vi "Create Image Name.vi"(8 "error in (no error)":errorcluster, 11 "Save Image in":refnum<class "Save Image.lvclass">) -> (0 "error out":errorcluster, 3 "Save Image out":refnum<class "Save Image.lvclass">)   [LabVIEW 2018, in "Save Image.lvclass"]
uses:
  Save Image.lvclass
  Save Image.lvclass/Save Image.ctl
  Simulated_Header/Simulated_Header.lvclass
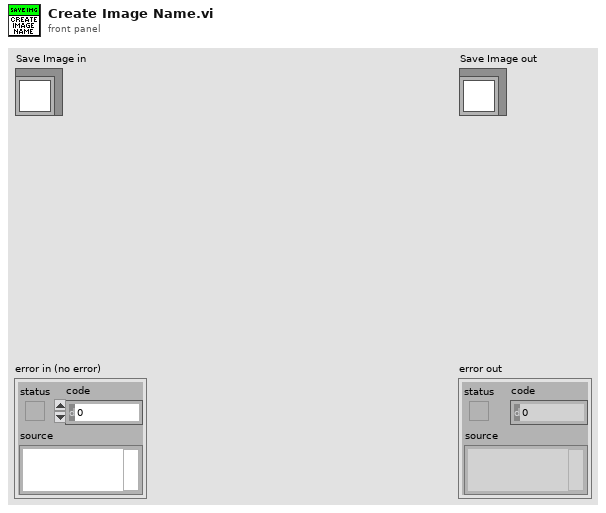
[diagram p1: front panel]
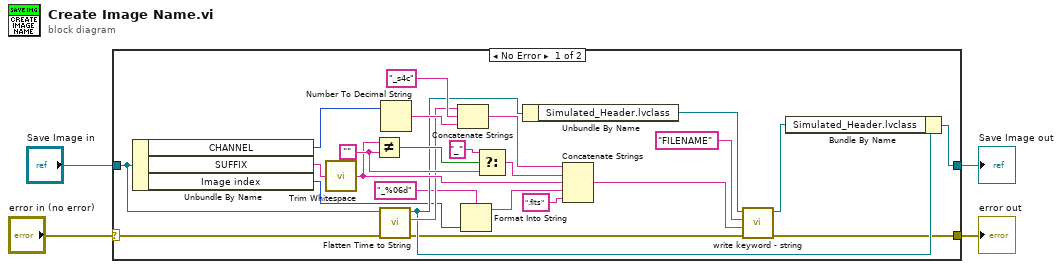
[diagram p0: block diagram]
diagram:
  n1 = case shown="No Error" "error in (no error)" {
    selector: "error in (no error)" -> [w18 w31]
    tunnel: [w9 w31] -> w3
    tunnel: [w15 w30] -> w1
    tunnel: "Save Image in" -> [w17 w30]
    frame No Error {
      w23 = ""
      n2 = Unbundle By Name(w17) -> ("CHANNEL"=w20:u16, "SUFFIX"=w22:string, "Image index"=w13:u32)
      n3 = call <vilib>:"Trim Whitespace.vi"("string"=w22) -> ("trimmed string"=w21:string)  [unwired: 1 in]
      n4 = Not Equal?(x=w21, y=w23) -> (x != y?=w26:bool)
      n5 = call "Flatten Time to String.vi"("error in (no error)"=w18, "Save Image in"=w17) -> ("error out"=w8:errorcluster, "flattened string"=w19:string, "Save Image out"=w16:refnum<class "Save Image.lvclass">)  [unwired: 7 in]
      n6 = Number To Decimal String(number=w20) -> (decimal integer string=w28:string)  [unwired: 1 in]
      n7 = Concatenate Strings(w19, "_s4c" ("string"), w28) -> (w27:string)
      n8 = Format Into String(format string="_%06d", w13) -> (resulting string=w12:string)  [unwired: 2 in, 1 out]
      n9 = Select(t="_" ("string"), s=w26, f=w23) -> (s? t:f=w24:string)
      n10 = Unbundle By Name(w16) -> ("Simulated_Header.lvclass"=w7:refnum<class "Simulated_Header.lvclass">)
      n11 = Concatenate Strings(w27, w24, w21, w12, ".fits" ("string")) -> (w6:string)
      n12 = call "write keyword - string.vi"("error in (no error)"=w8, "value"=w6, "keyword"="FILENAME", "Simulated_Header in"=w7) -> ("error out"=w9:errorcluster, "Simulated_Header out"=w10:refnum<class "Simulated_Header.lvclass">)  [unwired: 6 in]
      n13 = Bundle By Name(cluster=w16, "Simulated_Header.lvclass"=w10) -> (w15:refnum<class "Save Image.lvclass">)
    }
    frame Error {
    }
  }
  "error out" <- w3
  "Save Image out" <- w1
